vi "Lift Encoder.vi"(1 "Reset":bool, 2 "Mode":enum8{"Start", "Run", "Finish"}(ring)) -> (0 "Lift Encoder":T1)   [LabVIEW 2014]
uses:
  <vilib>/Rock Robotics/SystemInterfaces/DIO/FPGA_DIOChannel.ctl
  <vilib>/Rock Robotics/WPI/Counter/WPI_CounterDigitalInputToDigitalSource.vi
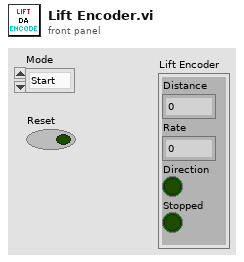
[diagram p1: front panel]
types:
  T1 = cluster{"Distance":dbl, "Rate":dbl, "Direction":bool, "Stopped":bool}
  T2 = typedef "FPGA_DIOChannel.ctl" = enum8{"DIO 0", "DIO 1", "DIO 2", "DIO 3", "DIO 4", "DIO 5", "DIO 6", "DIO 7", "DIO 8", "DIO 9", "DIO MXP 0", "DIO MXP 1", "DIO MXP 2", "DIO MXP 3", "DIO MXP 4", "DIO MXP 5", "DIO MXP 6", "DIO MXP 7", "DIO MXP 8", "DIO MXP 9", "DIO MXP 10", "DIO MXP 11", "DIO MXP 12", "DIO MXP 13", "DIO MXP 14", "DIO MXP 15", "Invalid"}
  T3 = typedef "WPI_EncoderDevRef.ctl" = cluster{"DevStatus":errorcluster, "EncoderIndex":T4, "CounterIndex":T5, "DistancePerCount":dbl, "Decoding Type":T6}
  T4 = typedef "FPGA_EncoderIdx.ctl" = enum8{"Enc 0", "Enc 1", "Enc 2", "Enc 3", "Enc 4", "Enc 5", "Enc 6", "Enc 7", "Invalid"}
  T5 = typedef "FPGA_CounterCtrSystemIndex.ctl" = enum8{"Ctr 0", "Ctr 1", "Ctr 2", "Ctr 3", "Ctr 4", "Ctr 5", "Ctr 6", "Ctr 7", "Invalid"}
  T6 = typedef "WPI_EncoderType.ctl" = enum16{"1x", "2x", "4x"}
  T7 = typedef "WPI_DigitalInputDevRef.ctl" = cluster{"DevStatus":errorcluster, "DIO Channel":T2, "Controller":T8}
  T8 = typedef "FPGA_TypedefDigitalModule.ctl" = enum16{"Controller 1"}
  T9 = typedef "FPGA_CounterEncoderSourceConvertionLVSourceType.ctl" = cluster{"DevStatus":errorcluster, "AnalogTriggerMode?":bool, "DigitalMode":cluster{"Controller":T8, "DIO Channel":T10}, "AnalogTriggerMode":cluster{"AnalogTriggerIndex":T11, "OutputType":T12}}
  T10 = typedef "FPGA_DIODigitalSourceChannel.ctl" = enum8{"DIO 0", "DIO 1", "DIO 2", "DIO 3", "DIO 4", "DIO 5", "DIO 6", "DIO 7", "DIO 8", "DIO 9", "DIO MXP 0", "DIO MXP 1", "DIO MXP 2", "DIO MXP 3", "DIO MXP 4", "DIO MXP 5", "DIO MXP 6", "DIO MXP 7", "DIO MXP 8", "DIO MXP 9", "DIO MXP 10", "DIO MXP 11", "DIO MXP 12", "DIO MXP 13", "DIO MXP 14", "DIO MXP 15", "Disabled"}
  T11 = typedef "FPGA_AnalogTriggerIndex.ctl" = enum8{"Trig 0", "Trig 1", "Trig 2", "Trig 3", "Trig 4", "Trig 5", "Trig 6", "Trig 7", "Invalid"}
  T12 = typedef "FPGA_AnalogTriggerOutType.ctl" = enum16{"InWindow", "TriggerState", "Rising", "Falling"}
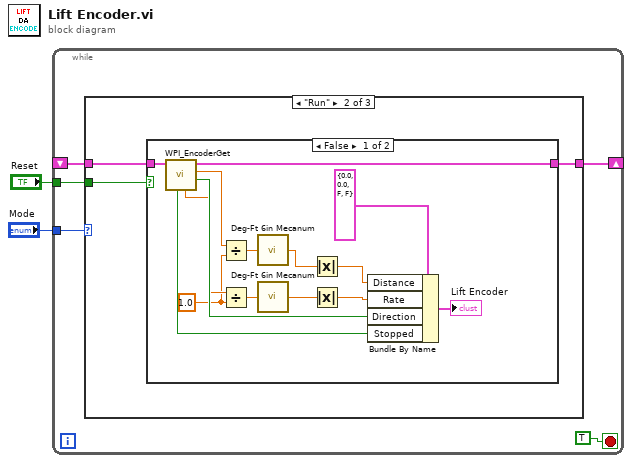
[diagram p0: block diagram]
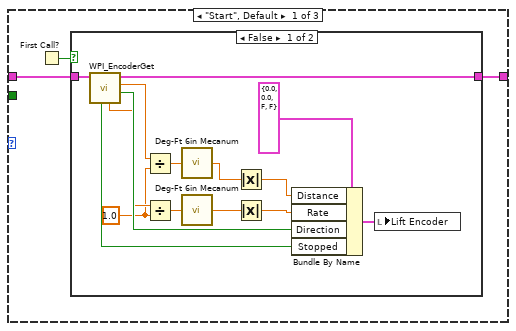
[diagram p2: hidden frame]
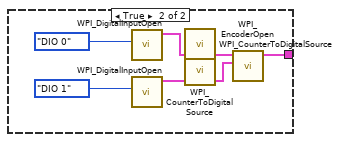
[diagram p3: hidden frame]
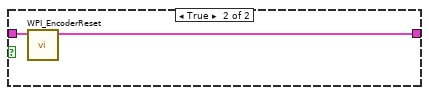
[diagram p4: hidden frame]
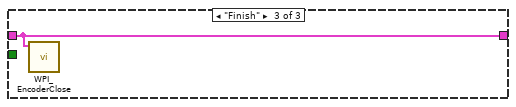
[diagram p5: hidden frame]
diagram:
  n1 = while {
    tunnel: "Mode" -> [w7]
    tunnel: "Reset" -> [w5]
    shift-right: [w4] -> _
    shift-left: _ -> [w3]
    stop <- TRUE stop-if-true
    n2 = case shown="\"Run\"" w7 {
      tunnel: w5 -> [_ w35 _]
      tunnel: [w9 w33 w53] -> w4
      tunnel: w3 -> [w8 w34 w53]
      frame "Start", Default {
        n3 = First Call?() -> (First Call?: T/F=w10:bool)
        n4 = case shown="False" w10 {
          tunnel: [w12 w26] -> w9
          tunnel: w8 -> [w13 _]
          frame False {
            w20 = 1.0 ("y")
            n5 = call <vilib>:"WPI_EncoderGet.vi"("EncoderDevRef"=w13) -> ("Direction"=w24:bool, "Distance"=w22:dbl, "EncoderDevRef"=w12:T3, "Rate"=w21:dbl, "Stopped"=w23:bool)  [unwired: 5 in, 1 out]
            n6 = Divide(x=w22, y=w20) -> (x/y=w18:dbl)
            n7 = Divide(x=w21, y=w20) -> (x/y=w19:dbl)
            n8 = call "Deg-Ft 6in Mecanum.vi"("Degrees"=w18) -> ("Feet"=w17:dbl)
            n9 = call "Deg-Ft 6in Mecanum.vi"("Degrees"=w19) -> ("Feet"=w16:dbl)
            n10 = Absolute Value(x=w17) -> (abs(x)=w15:dbl)
            n11 = Absolute Value(x=w16) -> (abs(x)=w14:dbl)
            n12 = Bundle By Name(cluster=T1 {"Distance"=0.0, "Rate"=0.0, "Direction"=FALSE, "Stopped"=FALSE} ("Encoder"), "Distance"=w15, "Rate"=w14, "Direction"=w24, "Stopped"=w23) -> (w11:T1)
            n13 = local write "Lift Encoder"(w11) -> ()
          }
          frame True {
            n14 = call <vilib>:"WPI_DigitalInputOpen.vi"("DIO Channel"=FPGA_DIOChannel."DIO 0") -> ("DigitalInputDevRef"=w30:T7)  [unwired: 2 in, 8 out]
            n15 = call <vilib>:"WPI_DigitalInputOpen.vi"("DIO Channel"=FPGA_DIOChannel."DIO 1") -> ("DigitalInputDevRef"=w31:T7)  [unwired: 2 in, 8 out]
            n16 = call-poly <vilib>:"WPI_CounterToDigitalSource.vi"("DigitalInputDevRef"=w30) -> ("Digital Source"=w29:T9)  [unwired: 6 out]
            n17 = call-poly <vilib>:"WPI_CounterToDigitalSource.vi"("DigitalInputDevRef"=w31) -> ("Digital Source"=w32:T9)  [unwired: 6 out]
            n18 = call <vilib>:"WPI_EncoderOpen.vi"("BSource"=w32, "ASource"=w29) -> ("EncoderDevRef"=w26:T3)  [unwired: 6 in, 3 out]
          }
        }
      }
      frame "Run" {
        n19 = case shown="False" w35 {
          tunnel: w34 -> [w38 w52]
          tunnel: [w37 w51] -> w33
          frame False {
            w45 = 1.0 ("y")
            n20 = call <vilib>:"WPI_EncoderGet.vi"("EncoderDevRef"=w38) -> ("Direction"=w49:bool, "Distance"=w47:dbl, "EncoderDevRef"=w37:T3, "Rate"=w46:dbl, "Stopped"=w48:bool)  [unwired: 5 in, 1 out]
            n21 = Divide(x=w47, y=w45) -> (x/y=w43:dbl)
            n22 = Divide(x=w46, y=w45) -> (x/y=w44:dbl)
            n23 = call "Deg-Ft 6in Mecanum.vi"("Degrees"=w43) -> ("Feet"=w42:dbl)
            n24 = call "Deg-Ft 6in Mecanum.vi"("Degrees"=w44) -> ("Feet"=w41:dbl)
            n25 = Absolute Value(x=w42) -> (abs(x)=w40:dbl)
            n26 = Absolute Value(x=w41) -> (abs(x)=w39:dbl)
            n27 = Bundle By Name(cluster=T1 {"Distance"=0.0, "Rate"=0.0, "Direction"=FALSE, "Stopped"=FALSE} ("Encoder"), "Distance"=w40, "Rate"=w39, "Direction"=w49, "Stopped"=w48) -> (→"Lift Encoder":T1)
          }
          frame True {
            n28 = call <vilib>:"WPI_EncoderReset.vi"("EncoderDevRef"=w52) -> ("EncoderDevRef"=w51:T3)  [unwired: 9 in, 1 out]
          }
        }
      }
      frame "Finish" {
        n29 = call <vilib>:"WPI_EncoderClose.vi"("EncoderDevRef"=w53) -> ()  [unwired: 10 in, 1 out]
      }
    }
  }
